vi "User select_listbox.vi"(6 "리스트명":string, 8 "error in":errorcluster caption="에러 입력(에러 없음)", 9 "Col Header in":string[](array[string]), 10 "Data in":string[][](array[string]), 11 "Func in":string) -> (0 "error out":errorcluster caption="에러 출력", 1 "배열":string[](array[string]), 2 "Text out":string, 3 "Func out":string)   [LabVIEW 2020]
uses:
  Controls/Cmd_User select.ctl
  Variables/Global_Cal Info.vi
  Polymorph/Cell Space_ListBox.vi
panel:
  in  "Select":i32(listbox) caption="전기 마이크로미터 Range 선택"
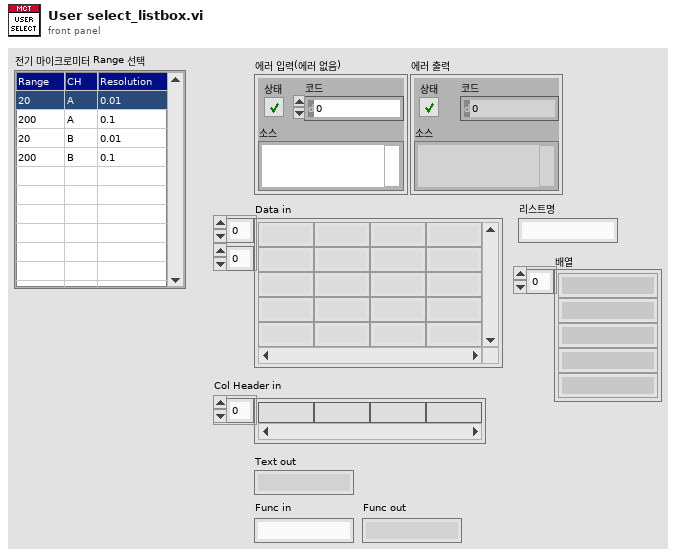
[diagram p1: front panel]
types:
  T1 = typedef "Cmd_User select.ctl" = enum16{"Initialize", "Command", "Exit"}
  T2 = enum32{"Invalid", "Default", "Floating", "Floating/Auto-Hide", "Modal"}
  T3 = typedef "LVBoundsTypeDef.ctl" = cluster{"Width":u32, "Height":u32}
  T4 = typedef "LVRectTypeDef.ctl" = cluster{"Left":i16, "Top":i16, "Right":i16, "Bottom":i16}
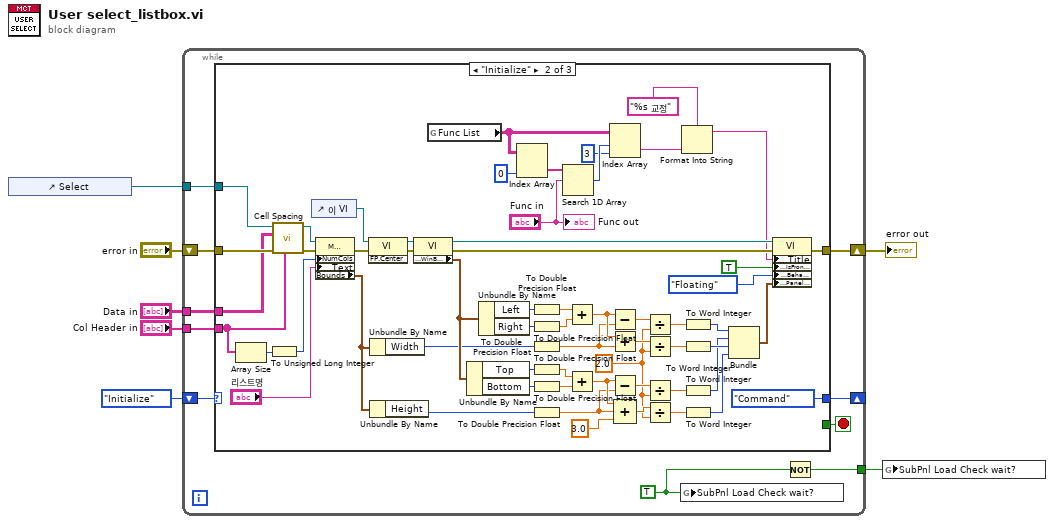
[diagram p0: block diagram]
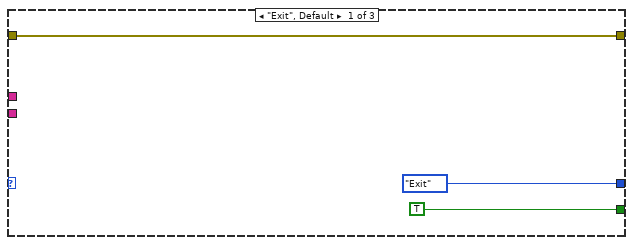
[diagram p2: hidden frame]
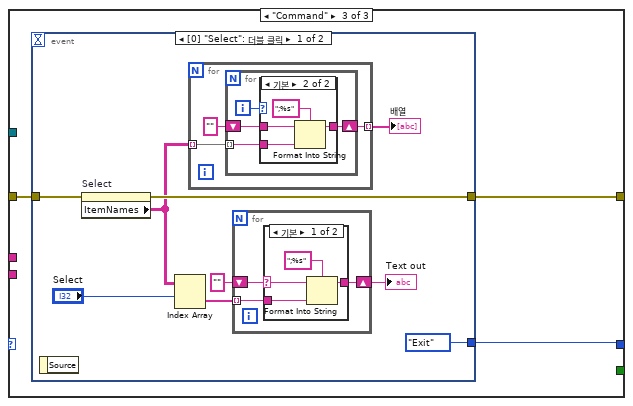
[diagram p3: hidden frame]
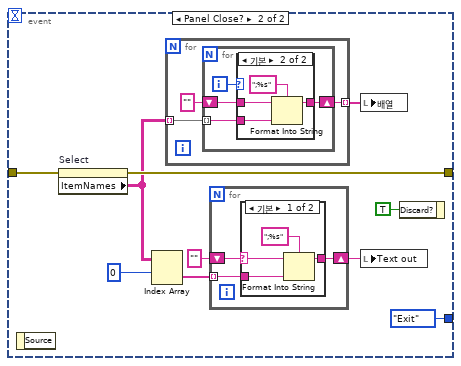
[diagram p6: hidden frame]
diagram:
  n1 = control-ref of="Select"() -> (w3:refnum<vi>)
  n2 = while {
    shift-right: [w12] -> _
    shift-left: Cmd_User_select."Initialize" -> [w17]
    tunnel: "Data in" -> [w16]
    shift-right: [w14] -> w5
    shift-left: "error in" -> [w15]
    tunnel: "Col Header in" -> [w13]
    tunnel: w3 -> [w10]
    tunnel: [w8] -> w1
    stop <- w11 stop-if-true
    w9 = TRUE ("SubPnl Load Check wait?")
    n3 = case shown="\"Initialize\"" w17 {
      tunnel: w16 -> [_ w74 _]
      tunnel: w15 -> [w19 w78 w81]
      tunnel: [w19 w69 w80] -> w14
      tunnel: w13 -> [_ w73 _]
      tunnel: [Cmd_User_select."Exit" Cmd_User_select."Command" w79] -> w12
      tunnel: [TRUE _ _] -> w11
      tunnel: w10 -> [_ w35 _]
      frame "Exit", Default {
      }
      frame "Initialize" {
        w49 = 2.0 ("y")
        n4 = Array Size(array=w73) -> (size(s)=w72:i32)
        n5 = To Unsigned Long Integer(number=w72) -> (unsigned 32bit integer=w71:u32)
        n6 = call-poly "Cell Spacing.vi"("Col Header in"=w73, "error in"=w78, "Data in"=w74, "여러열리스트박스 참조 in"=w35) -> ("error out"=w76:errorcluster, "여러열리스트박스 참조 out"=w75:refnum<vi>)  [unwired: 6 in]
        n7 = control-ref of="이 VI"() -> (w67:refnum<vi>)
        n8 = property class="MCListbox"(reference=w75, error in=w76, "NumCols"=w71, "Caption.Text"="리스트명") -> (error out=w66:errorcluster, "Bounds"=w37:T3)  [unwired: 1 out]
        n9 = invoke class="VI" method="FP.Center"(reference=w67, error in=w66) -> (reference out=w65:refnum<vi>, error out=w64:errorcluster)  [unwired: 1 in, 1 out]
        n10 = Unbundle By Name(w37) -> ("Width"=w36:u32)
        n11 = Unbundle By Name(w37) -> ("Height"=w51:u32)
        n12 = property on="프로퍼티 노드" class="VI"(reference=w65, error in=w64) -> (error out=w63:errorcluster, "Front Panel.WinBounds"=w38:T4)  [unwired: 1 out]
        n13 = global read "Global_Cal Info.vi" "Func List"() -> (w30:string[][])
        n14 = Unbundle By Name(w38) -> ("Top"=w40:i16, "Bottom"=w39:i16)
        n15 = Unbundle By Name(w38) -> ("Left"=w62:i16, "Right"=w61:i16)
        n16 = Index Array(array=w30, index (col)=0 ("비활성화된 인덱스 (열)")) -> (element=w28:string[])  [unwired: 1 in]
        n17 = To Double Precision Float(number=w62) -> (double precision float=w47:dbl)
        n18 = To Double Precision Float(number=w61) -> (double precision float=w46:dbl)
        n19 = To Double Precision Float(number=w36) -> (double precision float=w42:dbl)
        n20 = To Double Precision Float(number=w40) -> (double precision float=w45:dbl)
        n21 = To Double Precision Float(number=w39) -> (double precision float=w44:dbl)
        n22 = To Double Precision Float(number=w51) -> (double precision float=w41:dbl)
        n23 = Search 1D Array(1D array=w28, element="Func in") -> (index of element=w31:i32)  [unwired: 1 in]
        n24 = Add(x=w47, y=w46) -> (x+y=w55:dbl)
        n25 = Add(x=w45, y=w44) -> (x+y=w52:dbl)
        n26 = Index Array(array=w30, index (row)=w31, index (col)=3 ("비활성화된 인덱스 (열)")) -> (element=w23:string)
        n27 = Subtract(x=w55, y=w42) -> (x-y=w60:dbl)
        n28 = Add(x=w55, y=w42) -> (x+y=w59:dbl)
        n29 = Subtract(x=w52, y=w41) -> (x-y=w54:dbl)
        n30 = Compound Arithmetic op=ADD(w52, w41, 3.0 ("값")) -> (w50:dbl)
        n31 = Divide(x=w60, y=w49) -> (x/y=w58:dbl)
        n32 = Divide(x=w59, y=w49) -> (x/y=w57:dbl)
        n33 = Divide(x=w54, y=w49) -> (x/y=w53:dbl)
        n34 = Divide(x=w50, y=w49) -> (x/y=w48:dbl)
        n35 = Format Into String(format string="%s 교정" ("포맷 문자열"), w23) -> (resulting string=w24:string)  [unwired: 2 in, 1 out]
        n36 = To Word Integer(number=w58) -> (16bit integer=w43:i16)
        n37 = To Word Integer(number=w57) -> (16bit integer=w34:i16)
        n38 = To Word Integer(number=w53) -> (16bit integer=w33:i16)
        n39 = To Word Integer(number=w48) -> (16bit integer=w32:i16)
        n40 = Bundle(w43, w33, w34, w32) -> (w56:cluster{i16, i16, i16, i16})  [unwired: 1 in]
        n41 = property on="프로퍼티 노드" class="VI"(reference=w65, error in=w63, "Front Panel.Title"=w24, "Front Panel.IsFrontmost"=TRUE ("프런트패널 윈도우:맨 앞으로"), "FP.Behavior"=T2."Floating" ("프런트패널 윈도우:동작"), "Front Panel.PanelBounds"=w56) -> (error out=w69:errorcluster)  [unwired: 1 out]
        "Func out" <- "Func in"
      }
      frame "Command" {
        n42 = event shown="[0] \"Select\": 더블 클릭" {
          selector: _ -> [_ _]
          dyn-events: _ -> [_ _]
          timeout: _ -> [_ _]
          tunnel: w81 -> [w90 w116]
          tunnel: [w89 w114] -> w80
          tunnel: [Cmd_User_select."Exit" Cmd_User_select."Exit"] -> w79
          event "Select": Double Click {
            n43 = event-data() -> ()  [unwired: 1 in, 1 out]
            n44 = property on="Select" class="MCListbox (엄격한)"(error in=w90) -> (error out=w89:errorcluster, "ItemNames"=w82:string[][])  [unwired: 1 in, 1 out]
            n45 = Index Array(array=w82, index (row)="Select") -> (element=w87:string[])  [unwired: 1 in]
            n46 = for {
              tunnel: w82 -> [w93] mode=indexing
              tunnel: [w91] -> w83 mode=indexing
              n47 = for {
                tunnel: w93 -> [w95] mode=indexing
                shift-right: [w96] -> w91
                shift-left: "" -> [w97]
                i -> [w94]
                n48 = case shown="기본" w94 {
                  tunnel: w97 -> [_ w102]
                  tunnel: [w98 w101] -> w96
                  tunnel: w95 -> [w98 w100]
                  frame 0 {
                  }
                  frame Default {
                    n49 = Format Into String(format string=";%s" ("포맷 문자열"), initial string=w102, w100) -> (resulting string=w101:string)  [unwired: 1 in, 1 out]
                  }
                }
              }
            }
            "배열" <- w83
            n50 = for {
              tunnel: w87 -> [w103] mode=indexing
              shift-right: [w104] -> w85
              shift-left: "" -> [w105]
              n51 = case shown="기본" w105 {
                selector: w105 -> [w108 _]
                tunnel: [w107 w110] -> w104
                tunnel: w103 -> [w109 w110]
                frame Default {
                  n52 = Format Into String(format string=";%s" ("포맷 문자열"), initial string=w108, w109) -> (resulting string=w107:string)  [unwired: 1 in, 1 out]
                }
                frame "" {
                }
              }
            }
            "Text out" <- w85
          }
          event Panel Close? {
            n53 = event-data() -> ()  [unwired: 1 in, 1 out]
            n54 = property on="Select" class="MCListbox (엄격한)"(error in=w116) -> (error out=w114:errorcluster, "ItemNames"=w112:string[][])  [unwired: 1 in, 1 out]
            n55 = Index Array(array=w112, index (row)=0 ("인덱스 (행)")) -> (element=w118:string[])  [unwired: 1 in]
            n56 = for {
              tunnel: w112 -> [w123] mode=indexing
              tunnel: [w121] -> w111 mode=indexing
              n57 = for {
                tunnel: w123 -> [w125] mode=indexing
                shift-right: [w126] -> w121
                shift-left: "" -> [w127]
                i -> [w124]
                n58 = case shown="기본" w124 {
                  tunnel: w127 -> [_ w132]
                  tunnel: [w128 w131] -> w126
                  tunnel: w125 -> [w128 w130]
                  frame 0 {
                  }
                  frame Default {
                    n59 = Format Into String(format string=";%s" ("포맷 문자열"), initial string=w132, w130) -> (resulting string=w131:string)  [unwired: 1 in, 1 out]
                  }
                }
              }
            }
            n60 = for {
              tunnel: w118 -> [w133] mode=indexing
              shift-right: [w134] -> w113
              shift-left: "" -> [w135]
              n61 = case shown="기본" w135 {
                selector: w135 -> [w138 _]
                tunnel: [w137 w140] -> w134
                tunnel: w133 -> [w139 w140]
                frame Default {
                  n62 = Format Into String(format string=";%s" ("포맷 문자열"), initial string=w138, w139) -> (resulting string=w137:string)  [unwired: 1 in, 1 out]
                }
                frame "" {
                }
              }
            }
            n63 = local write "배열"(w111) -> ()
            n64 = local write "Text out"(w113) -> ()
            n65 = event-data("Discard?"=TRUE ("버림?")) -> ()  [unwired: 1 in, 1 out]
          }
        }
      }
    }
    n66 = global write "Global_Cal Info.vi" "SubPnl Load Check wait?"(w9) -> ()
    n67 = Not(x=w9) -> (.not. x?=w8:bool)
  }
  "error out" <- w5
  n68 = global write "Global_Cal Info.vi" "SubPnl Load Check wait?"(w1) -> ()
